vi "STM_Client_3.vi"() -> ()   [LabVIEW 2016]
uses:
  <vilib>/NI/STM/SubVIs/MetaDataElement.ctl
  RemoteControl/Typedefs/Variant with Message ID--cluster.ctl
  <vilib>/NI/STM/TCP/Read Meta Data (TCP Ref).vi
  <vilib>/NI/STM/TCP/Get Connection Reference (TCP).vi
  <vilib>/NI/STM/TCP/Read Meta Data (TCP Clst).vi
  <userlib>/_OpenG.lib/numeric/numeric.llb/Random Number Within Range - I32__ogtk.vi
  <vilib>/NI/STM/TCP/Write Message (TCP).vi
  <vilib>/NI/STM/TCP/Read Message (TCP).vi
  <userlib>/_OpenG.lib/error/error.llb/Filter Error Codes (Array)__ogtk.vi
  <vilib>/NI/STM/NI STM.lvlib
  RemoteControl/RemoteControl.lvclass
panel:
  out "Numeric":i32
  out "value":i32
  out "messsages/s":dbl
  in  "stop":bool
  out "reponse command":string
  out "response data":string
  out "setMagnet":dbl
  out "unknown":string
  out "HELP":string[](array[string])
  in  "Command":string
  out "duration ms":u32
  in  "remote address":string
  out "meta data\n(available commands)":T1[](array[typedef])
  out "ACK":string
  in  "data to send":dbl
  out "error out":errorcluster
  # "CLIENT (API)"
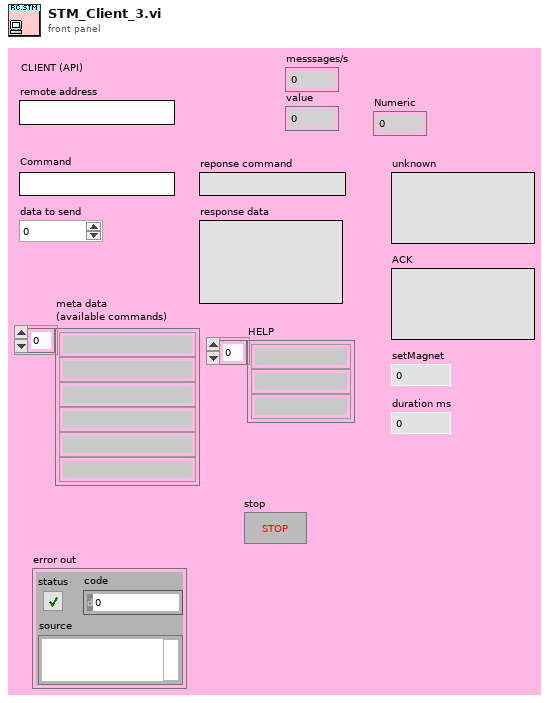
[diagram p1: front panel]
types:
  T1 = typedef "NI STM.lvlib/MetaDataElement.ctl" = string
  T2 = typedef "RemoteControl.lvclass/Variant with Message ID--cluster.ctl" = cluster{"Data":variant, "Message ID":i32}
  T3 = typedef "NI STM.lvlib/TCP Connection Info.ctl" = cluster{"connection ID":refnum<k5>, "meta data":T1[]}
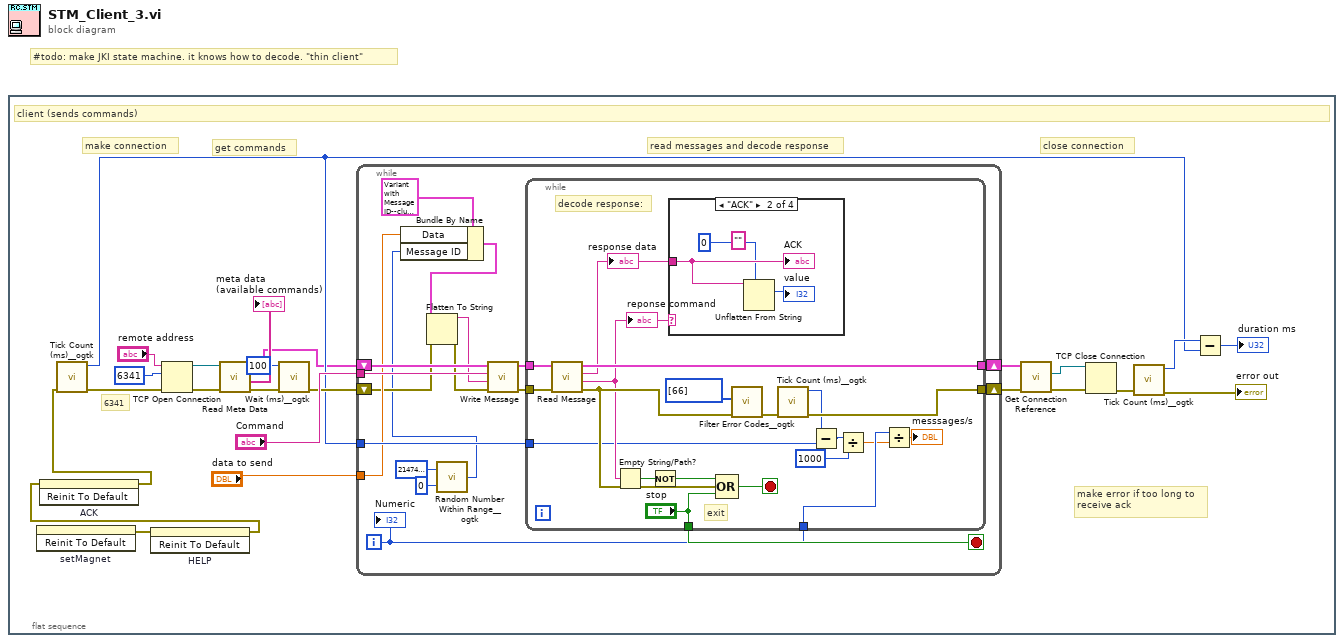
[diagram p0: block diagram]
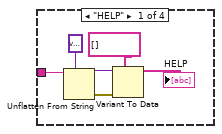
[diagram p2: hidden frame]
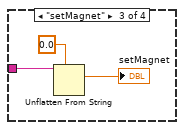
[diagram p3: hidden frame]
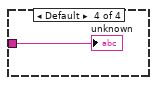
[diagram p4: hidden frame]
diagram:
  # "#todo: make JKI state machine. it knows how to decode. \"thin client\""
  n1 = flat-sequence {
    frame #0 {
      # "close connection"
      # "read messages and decode response"
      # "get commands"
      # "make connection"
      # "6341"
      # "make error if too long to\nreceive ack"
      # "client (sends commands)"
      n2 = invoke on="setMagnet" class="DigNum (strict)" method="Reinit To Default"() -> (error out=w11:errorcluster)  [unwired: 3 in, 2 out]
      n3 = invoke on="HELP" class="Arr (strict)" method="Reinit To Default"(error in=w11) -> (error out=w10:errorcluster)  [unwired: 2 in, 2 out]
      n4 = invoke on="ACK" class="Str" method="Reinit To Default"(error in=w10) -> (error out=w12:errorcluster)  [unwired: 2 in, 2 out]
      n5 = call <userlib>:"Tick Count (ms)__ogtk.vi"("error in (no error)"=w12) -> ("error out"=w19:errorcluster, "millisecond timer value"=w3:u32)  [unwired: 9 in]
      n6 = TCP Open Connection(address="remote address", remote port or service name=u16 6341, error in (no error)=w19) -> (connection ID=w23:refnum<k5>, error out=w24:errorcluster)  [unwired: 2 in]
      n7 = call-poly <vilib>:"Read Meta Data.vi"("error in"=w24, "connection ID"=w23) -> ("error out"=w6:errorcluster, "meta data"=→"meta data\n(available commands)":T1[], "connection info out"=w1:T3)  [unwired: 7 in]
      n8 = call <userlib>:"Wait (ms)__ogtk.vi"("error in (no error)"=w6, "milliseconds to wait"=u32 100) -> ("error out"=w5:errorcluster)  [unwired: 8 in, 1 out]
      n9 = while {
        tunnel: "Command" -> [w38]
        shift-right: [w40] -> w18
        shift-left: w5 -> [w30]
        shift-right: [w39] -> w17
        shift-left: w1 -> [w37]
        tunnel: w3 -> [w35]
        tunnel: "data to send" -> [w32]
        i -> [w33]
        stop <- w36 stop-if-true
        n10 = call-poly <userlib>:"Random Number Within Range__ogtk.vi"("High"=2147483647, "Low"=0) -> ("Random Number"=w25:i32)  [unwired: 3 in]
        n11 = Bundle By Name(cluster=T2 {"Data"=variant, "Message ID"=0} ("output cluster"), "Data"=w32, "Message ID"=w25) -> (w31:T2)
        n12 = Flatten To String(anything=w31, error in (no error)=w30) -> (data string=w29:string, error out=w28:errorcluster)  [unwired: 2 in, 1 out]
        n13 = call-poly <vilib>:"Write Message.vi"("error in"=w28, "data"=w29, "name"=w38, "connection info in"=w37) -> ("error out"=w42:errorcluster, "connection info out"=w41:T3)  [unwired: 6 in]
        n14 = while {
          tunnel: w42 -> [w62]
          tunnel: w41 -> [w61]
          tunnel: [w50] -> w40
          tunnel: [w60] -> w39
          tunnel: ["stop"] -> w36
          tunnel: w35 -> [w48]
          tunnel: w33 -> [w45]
          stop <- w59 stop-if-true
          # "decode response:"
          # "exit"
          n15 = call-poly <vilib>:"Read Message.vi"("error in"=w62, "connection info in"=w61) -> ("error out"=w58:errorcluster, "name"=w55:T1, "data string"=w56:string, "connection info out"=w60:T3)  [unwired: 2 in, 4 out]
          "response data" <- w56
          "reponse command" <- w55
          n16 = Empty String/Path?(string/path=w55) -> (empty?=w54:bool)
          n17 = Not(x=w54) -> (.not. x?=w53:bool)
          n18 = case shown="\"ACK\"" w55 {
            tunnel: w56 -> [w68 w71 w74 w75]
            frame "HELP" {
              n19 = Unflatten From String(type=variant, binary string=w68) -> (value=w65:variant, error out=w66:errorcluster)  [unwired: 3 in, 1 out]
              n20 = Variant To Data(error in=w66, type=string[] [] ("HELP"), Variant=w65) -> (data=→"HELP":string[])  [unwired: 1 out]
            }
            frame "ACK" {
              (unwired) ""
              n21 = Unflatten From String(type=0, binary string=w71) -> (value=→"value":i32)  [unwired: 3 in, 2 out]
              "ACK" <- w71
            }
            frame "setMagnet" {
              n22 = Unflatten From String(type=0.0, binary string=w74) -> (value=→"setMagnet":dbl)  [unwired: 3 in, 2 out]
            }
            frame Default {
              "unknown" <- w75
            }
          }
          n23 = Compound Arithmetic op=OR(w53, w58, "stop") -> (w59:bool)
          n24 = call-poly <userlib>:"Filter Error Codes__ogtk.vi"("Error In"=w58, "Error Codes to Filter"=i32[] [66]) -> ("Error Out"=w51:errorcluster)  [unwired: 7 in, 2 out]
          n25 = call <userlib>:"Tick Count (ms)__ogtk.vi"("error in (no error)"=w51) -> ("error out"=w50:errorcluster, "millisecond timer value"=w49:u32)  [unwired: 9 in]
          n26 = Subtract(x=w49, y=w48) -> (x-y=w47:u32)
          n27 = Divide(x=w47, y=u32 1000) -> (x/y=w44:dbl)
          n28 = Divide(x=w45, y=w44) -> (x/y=→"messsages/s":dbl)
        }
        "Numeric" <- w33
      }
      n29 = call-poly <vilib>:"Get Connection Reference.vi"("error in"=w18, "connection info in"=w17) -> ("error out"=w21:errorcluster, "connection ID out"=w20:refnum<k5>)  [unwired: 7 in, 1 out]
      n30 = TCP Close Connection(connection ID=w20, error in (no error)=w21) -> (error out=w16:errorcluster)  [unwired: 1 in, 1 out]
      n31 = call <userlib>:"Tick Count (ms)__ogtk.vi"("error in (no error)"=w16) -> ("error out"=→"error out":errorcluster, "millisecond timer value"=w13:u32)  [unwired: 9 in]
      n32 = Subtract(x=w13, y=w3) -> (x-y=→"duration ms":u32)
    }
  }
